vi "AlliGator Run FLI Dataset Python Function (API v1.1).vi"(7 "AlliGator Ctrl Refnums":T1, 8 "error in (no error)":errorcluster, 9 "Current Data":string, 10 "Python Function Info":T10={"Script Path"=path "", "Function Name"="", "Function Parent Menu"="", "API Version"="", "Function Input Parameters"=[], "Function Outputs"=[], "Function Doc String"="", "Function Display Name"="", "Function Target Type"=enum."Window Menu", "Function Target Window"="", "Parent Menu Location"="", "Item Menu Tag"="", "Is preceded by Separator"=FALSE}, 11 "Data Value Reference in":refnum<data-value>) -> (0 "error out":errorcluster, 1 "Message":string, 2 "Function Output Destination":string, 3 "Data Value Reference out":refnum<data-value>, 4 "Variant data out":variant)   [LabVIEW 2021, in "AlliGator Python Plugins.lvlib"]
doc: "Runs FLI Dataset python plugin function."
uses:
  AlliGator Python Plugins.lvlib
  Internal Variables/AlliGator Internal Variables v2.ctl
  <vilib>/vision/Image Controls.llb/IMAQ Image.ctl
  Internal Variables/AlliGator Gate Image Set.ctl
  Files/AlliGator FLI Dataset Type.ctl
  Files/AlliGator Data Series Type.ctl
  Dual-Channel Datasets/AlliGator Dataset Channel.ctl
  Settings/AlliGator Gate Arithmetic.ctl
  Source Image/AlliGator Displayed Image.ctl
  Image/Named ROI Description.ctl
  Phasor Graph/AlliGator Decay Metadata v3.ctl
  Decay Analysis/Decay Preprocessing/AlliGator Decay Background Subtraction Info.ctl
  Decay Analysis/Decay Preprocessing/AlliGator Baseline Subtraction Method.ctl
  Graphs/XY Graph/XY Graph Plot Shift Parameters.ctl
  Graphs/XY Graph/XY Graph Plot Shift Method.ctl
  Decay Analysis/Decay Preprocessing/AlliGator Decay Extrapolation Parameters.ctl
  Phasor/Calibration Phasor (m, phi).ctl
  Phasor/Phasor Reference Series.ctl
  Phasor/Phasor Calibration Map v2.ctl
  Phasor/Phasor (g, s).ctl
  Phasor Graph/AlliGator Raw Phasor Plot Data v5.ctl
  Phasor/Phasor Standard Deviation Options.ctl
  Phasor Plot/AlliGator Phasor Multi-Harmonic Data.ctl
  Phasor/Phasor Harmonic Data.ctl
  Decay Fit Parameter Map/AlliGator Decay Fit Options & Parameters v4.ctl
  Fits/IRF(X)PSED/Decay Fit Options v4.ctl
  Fits/Decay Convolution/Decay Model.ctl
  Fits/Residual Type.ctl
  Fits/IRF(X)PSED/Fit Weights Type v2.ctl
  Fits/Non-linear Fitting Method v2.ctl
  Fits/Fit Calculation Method.ctl
  Fits/Non-linear Fitting Algorithm.ctl
  Decay Analysis/Decay Fit/AlliGator Decay Fit Parameter Constraints 2.ctl
  Fits/IRF(X)PSED/Decay Fit Parameters In List.ctl
  Fits/IRF(X)PSED/MLE Baseline Offset Type.ctl
  Decay Analysis/Decay Preprocessing/AlliGator Decay Preprocessing Parameters.ctl
  Fits/IRF(X)PSED/Decay Fit Parameters & Derived Quantities List v2.ctl
  Fits/IRF(X)PSED/Decay Fit Result Constraint.ctl
  Decay Fit Parameter Map/AlliGator Parameter Maps Data.ctl
  AlliGator Python Function Information.ctl
  AlliGator Python Function Parameter Definition.ctl
  AlliGator Python Function Output Definition.ctl
  AlliGator Python Plugin Target Type.ctl
  Globals, Variables, Constants/AlliGator Variables List.ctl
  AlliGator Python Plugin Data v1.1.ctl
  API v1/AlliGator Python Plugin Image Data v1.ctl
  API v1/AlliGator Python Plugin Graph Data v1.ctl
  API v1/AlliGator Python Plugin Plot Data v1.ctl
  AlliGator Python Plugin Parameter Map Data v1.1.ctl
  Image/Image Point.ctl
  AlliGator Python Plugin FLI Dataset Data v1.1.ctl
  Parameter Map/AlliGator New Parameter Map Set Event Data.ctl
  <vilib>/Utility/error.llb/Error Cluster From Error Code.vi
  <vilib>/ErrorRing/Error Ring.xnode
  Globals, Variables, Constants/AlliGator Globals, Variables & Constants.lvlib
  Error/Error.lvlib
  Image/Image.lvlib
  Time/Time.lvlib
  Parameter Map/AlliGator Parameter Map.lvlib
  Strings/Strings.lvlib
  Phasor/Phasor.lvlib
  Decay Analysis/Decay Preprocessing/AlliGator Decay Preprocessing.lvlib
  Graphs/XY Graph/XY Graph Add-Ons.lvlib
  Phasor Graph/AlliGator Phasor Graph.lvlib
  Files/AlliGator Files.lvlib
  Phasor Plot/AlliGator Phasor Plot.lvlib
  Source Image/AlliGator Source Image.lvlib
  Fits/Fits.lvlib
  Decay Analysis/Decay Fit/AlliGator Decay Fit.lvlib
  Internal Variables/AlliGator Internal Variables.lvlib
  Settings/AlliGator Settings.lvlib
  Dual-Channel Datasets/AlliGator Dual-Channel Datasets.lvlib
  Decay Fit Parameter Map/AlliGator Decay Fit Parameter Map.lvlib
  GUI/AlliGator Registered Events Ctrl Refnums.ctl
  GUI/AlliGator GUI.lvlib
  GUI/AlliGator Dataset Ctrl Refnums.ctl
  Phasor/Phasor Calibration Type.ctl
  GUI/AlliGator Phasor Graph Ctrl Refnums.ctl
  GUI/AlliGator Phasor Plot Ctrl Refnums.ctl
  GUI/AlliGator State Indicator.ctl
  GUI/AlliGator Main Window Tabs.ctl
  GUI/AlliGator Other Ctrl Refnums.ctl
  Histograms/Histogram Bin Position.ctl
  Histograms/Histogram Window.lvlib
  Histograms/Histogram Bin Option.ctl
  Histograms/Linear Histogram Options.ctl
  GUI/AlliGator Image Histogram Control Refnums.ctl
  Decay Fit Parameter Map/AlliGator Decay Fit Map Control Refnums.ctl
  Parameter Map/AlliGator Parameter Map Control Refnums.ctl
  GUI/AlliGator Ctrl Refnums.ctl
panel:
  out "session out":refnum<k35>
  out "Function Parameters String":string
  # "see the AlliGator License on the block diagram (Ctrl+E or Window:Show Block Diagram)"
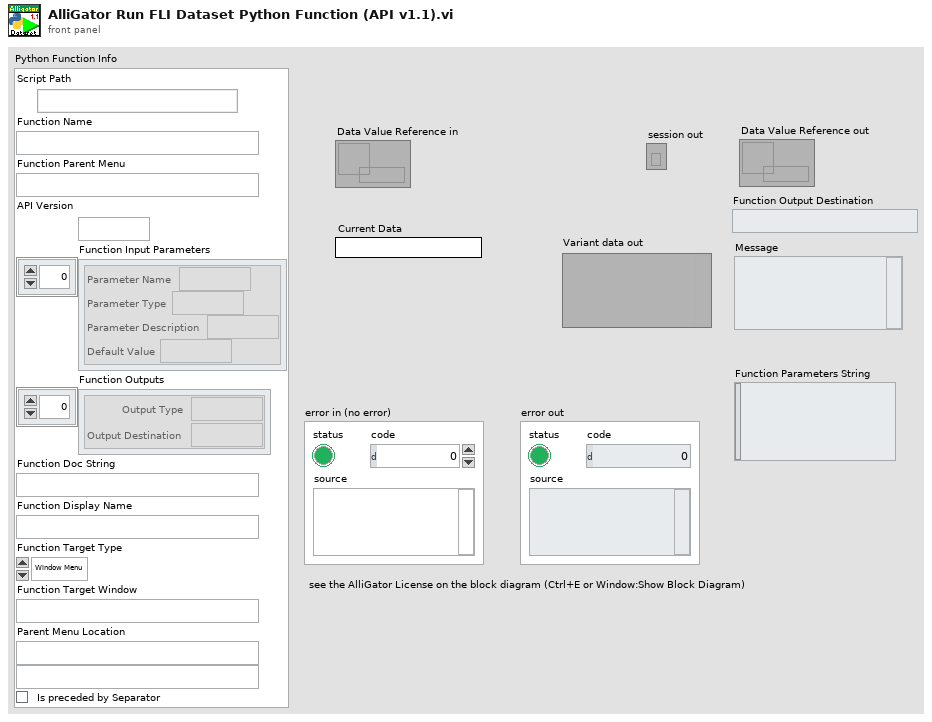
[diagram p1: front panel]
types:
  T1 = typedef "AlliGator GUI.lvlib/AlliGator Ctrl Refnums.ctl" = cluster{"Other AlliGator Ctrl Refnums":T2, "Phasor Plot Ctrl Refnums":T3, "Phasor Graph Ctrl Refnums":T4, "Dataset Control Refnums":T5, "Registered Events Ctrl Refnums":T6, "Image Histogram Ctrl Refnums":T7, "Decay Fit Map Ctrl Refnums":T8, "Parameter Map Ctrl Refnums":T9}
  T2 = typedef "AlliGator GUI.lvlib/AlliGator Other Ctrl Refnums.ctl" = cluster{"State Indicators":refnum<vi>, " Progress Bar":refnum<vi>, "Decay Graph Active":refnum<vi>, "Decay Statistics Bin":refnum<vi>, "Time Step":refnum<vi>, "Use File Timestamp":refnum<vi>, "Tab Control":refnum<vi>, "CPU":refnum<vi>, "Abort Fit":refnum<vi>, "Dataset File/Folder Path":refnum<vi>, "Abort ROI Creation":refnum<vi>, "Event LED":refnum<vi>, "Dataset File/Folder Path 2":refnum<vi>, "Dataset File/Folder Path 3":refnum<vi>, "Dataset File/Folder Path 4":refnum<vi>, "Dataset File/Folder Path 5":refnum<vi>, "Dataset File/Folder Path 6":refnum<vi>, "Dataset File/Folder Path 7":refnum<vi>, "Dataset File/Folder Path 8":refnum<vi>, "Dataset File/Folder Path 9":refnum<vi>, "Dataset File/Folder Path 10":refnum<vi>, "Dataset File/Folder Path 11":refnum<vi>}
  T3 = typedef "AlliGator GUI.lvlib/AlliGator Phasor Plot Ctrl Refnums.ctl" = cluster{"Phasor Ratio":refnum<vi>, "Modulus Lifetime":refnum<vi>, "Phasor at cursor (m, phi)":refnum<vi>, "Phase Lifetime":refnum<vi>, "Phasor at cursor (g, s)":refnum<vi>, "Phasor Plor Average Lifetime":refnum<vi>, "Phasor Plot Active":refnum<vi>, "Save Phasor Plot":refnum<vi>, "Image Overlay Color":refnum<vi>, "Phasor Plot Color Scale":refnum<vi>, "Reference 1 Button":refnum<vi>, "Reference 2 Button":refnum<vi>, "True Phasor Plot Value":refnum<vi>}
  T4 = typedef "AlliGator GUI.lvlib/AlliGator Phasor Graph Ctrl Refnums.ctl" = cluster{"Phasor Ratio":refnum<vi>, "Modulus Lifetime":refnum<vi>, "Phasor at cursor (m, phi)":refnum<vi>, "Phase Lifetime":refnum<vi>, "Phasor at cursor (g, s)":refnum<vi>, "Phasor Graph Average Lifetime":refnum<vi>, "Phasor Graph Active":refnum<vi>, "Save Phasor Graph":refnum<vi>, "Phasor Frame Slide":refnum<vi>, "Single Step Phasor":refnum<vi>, "Calibration Type":refnum<vi>, "Show Line":refnum<vi>, "Phase Lifetime 1":refnum<vi>, "Phase Lifetime 2":refnum<vi>, "Phasor Graph Frequency":refnum<vi>, "Phasor Reference 1 Control":refnum<vi>, "Phasor Reference 2 Control":refnum<vi>, "Calibration Lifetime":refnum<vi>, "Phase Lifetime SDV":refnum<vi>, "Average Lifetime SDV":refnum<vi>, "Phasor Ratio SDV":refnum<vi>, "Modulus Lifetime SDV":refnum<vi>}
  T5 = typedef "AlliGator GUI.lvlib/AlliGator Dataset Ctrl Refnums.ctl" = cluster{"Current Data":refnum<vi>, "Gate Image Slide":refnum<vi>, "Time Point Slide":refnum<vi>, "Current Time Stamp":refnum<vi>, "Save Image":refnum<vi>, "Displayed Image":refnum<vi>, "Overlay Mode":refnum<vi>, "Phasor Overlay Color":refnum<vi>, "Image Color Scale":refnum<vi>, "Use ROI as Search Area":refnum<vi>, "Source Image ROI Color":refnum<vi>, "True Pixel Value":refnum<vi>}
  T6 = typedef "AlliGator GUI.lvlib/AlliGator Registered Events Ctrl Refnums.ctl" = cluster{"Time Point Slider":refnum<vi>, "Phasor Plot Display Range":refnum<vi>, "Decay Graph":refnum<vi>, "Decay Statistics Graph":refnum<vi>, "Intensity Time Trace":refnum<vi>, "Phasor Graph":refnum<vi>, "Phasor Ratio Graph":refnum<vi>, "Lifetime Graph":refnum<vi>, "Phasor Plot Display":refnum<vi>, "Source Image Display":refnum<vi>, "Decay Fit Parameter Map Display Range":refnum<vi>, "Decay Fit Parameter Map Display":refnum<vi>, "Parameter Map Display Range":refnum<vi>, "Parameter Map Display":refnum<vi>, "Phasor Plot Display Range":refnum<vi>}
  T7 = typedef "AlliGator GUI.lvlib/AlliGator Image Histogram Control Refnums.ctl" = cluster{"Image Histogram":refnum<vi>, "Image Histogram Options":refnum<vi>, "Image Histogram Active":refnum<vi>, "Image Histogram Upper Percentile":refnum<vi>, "Image Histogram Lower Percentile":refnum<vi>, "Auto-Adjust Contrast":refnum<vi>}
  T8 = typedef "AlliGator Decay Fit Parameter Map.lvlib/AlliGator Decay Fit Map Control Refnums.ctl" = cluster{"Decay Fit Parameter Map Color Scale":refnum<vi>, "Decay Fit Parameter":refnum<vi>, "Max Parameter":refnum<vi>, "Min Parameter":refnum<vi>, "Decay Fit Parameter Map Display":refnum<vi>, "Decay Fit Parameter Map Display Range":refnum<vi>, "Decay Parameter Map X":refnum<vi>, "Decay Parameter Map Y":refnum<vi>, "Decay Parameter Map Value":refnum<vi>}
  T9 = typedef "AlliGator Parameter Map.lvlib/AlliGator Parameter Map Control Refnums.ctl" = cluster{"Parameter Map Color Scale":refnum<vi>, "Map Parameter":refnum<vi>, "Max Parameter":refnum<vi>, "Min Parameter":refnum<vi>, "Parameter Map Display":refnum<vi>, "Parameter Map Display Range":refnum<vi>, "Parameter Map Set":refnum<vi>, "Parameter Map X":refnum<vi>, "Parameter Map Y":refnum<vi>, "Parameter Map Value":refnum<vi>}
  T10 = typedef "AlliGator Python Plugins.lvlib/AlliGator Python Function Information.ctl" = cluster{"Script Path":path, "Function Name":string, "Function Parent Menu":string, "API Version":string, "Function Input Parameters":T11[], "Function Outputs":T12[], "Function Doc String":string, "Function Display Name":string, "Function Target Type":T13, "Function Target Window":string, "Parent Menu Location":string, "Item Menu Tag":string, "Is preceded by Separator":bool}
  T11 = typedef "AlliGator Python Plugins.lvlib/AlliGator Python Function Parameter Definition.ctl" = cluster{"Parameter Name":string, "Parameter Type":string, "Parameter Description":string, "Default Value":string}
  T12 = typedef "AlliGator Python Plugins.lvlib/AlliGator Python Function Output Definition.ctl" = cluster{"Output Type":string, "Output Destination":string}
  T13 = typedef "AlliGator Python Plugins.lvlib/AlliGator Python Plugin Target Type.ctl" = enum16{"Undefined", "Window Menu", "Object Menu"}
  T14 = typedef "AlliGator Python Plugins.lvlib/AlliGator Python Plugin Data v1.1.ctl" = cluster{"Image_Plugin_Data":T15, "Graph_Plugin_Data":T16, "Parameter_Map_Plugin_Data":T18, "FLI_Dataset_Plugin_Data":T20}
  T15 = typedef "AlliGator Python Plugins.lvlib/AlliGator Python Plugin Image Data v1.ctl" = cluster{"Image_Name":string, "Image":sgl[][]}
  T16 = typedef "AlliGator Python Plugins.lvlib/AlliGator Python Plugin Graph Data v1.ctl" = cluster{"Graph_Name":string, "Plots":T17[], "Reference_Decay":T17}
  T17 = typedef "AlliGator Python Plugins.lvlib/AlliGator Python Plugin Plot Data v1.ctl" = cluster{"Plot_Name":string, "X_Array":dbl[], "Y_Array":dbl[]}
  T18 = typedef "AlliGator Python Plugins.lvlib/AlliGator Python Plugin Parameter Map Data v1.1.ctl" = cluster{"Parameter_Names":string[], "Parameter_Flattened_Map":dbl[][], "Locations":T19[], "IRF_X":dbl[], "IRF_Y_Flattened_List":dbl[][], "X_Resolution":i32, "Y_Resolution":i32}
  T19 = typedef "Image.lvlib/Image Point.ctl" = cluster{"X":i32, "Y":i32}
  T20 = typedef "AlliGator Python Plugins.lvlib/AlliGator Python Plugin FLI Dataset Data v1.1.ctl" = cluster{"FLI_Dataset_Name":string, "Gate_Duration":dbl, "Gate_Separation":dbl, "Gate_Number":i32, "X_Size":i32, "Y_Size":i32, "Image_Data_List":T15[], "Mask_Image":u16[][], "Sum_Image":sgl[][], "Max_Image":sgl[][], "Min_Image":sgl[][]}
  T21 = typedef "AlliGator Globals, Variables & Constants.lvlib/AlliGator Variables List.ctl" = enum16{"---- GUI ----", "GUI:Initialization Status", "GUI:State Indicators Refnum", "GUI:Original AlliGator Menu Items", "GUI:Current Action Loop State", "GUI:Script in progress", "GUI:Playback", "GUI:Loop Playback", "GUI:Search ROI Used", "GUI:Search ROI", "Decay Graph Max Legend Size", "Intensity Graph Max Legend Size", "Decay Statistics Graph Max Legend Size", "Phasor Graph Max Legend Size", "Phasor Ratio Graph Max Legend Size", "Lifetime Graph Max Legend Size", "---- Files ----", "Files:Export Dataset Frames as Individual Files", "Files:Show Batch Export Help Balloons", "Files:Frames in Dataset", "Files:ptu File Frame Start Indices", "Files:Current Frame in Dataset", "Files:Current Frame Timestamp", "Files:Dataset Loaded", "Files:Dataset Metadata", "Files:Dataset Channel", "Files:Dataset Data Description", "Files:Background Dataset Metadata", "Files:Background Dataset Channel", "Files:Background Dataset Data Description", "Files:Background File Subtraction", "Files:Background File Path", "Files:Background File Pile-up Correction", "Files:Background File Pixel Well Capacity", "Files:Background File Scaling Factor", "Files:Current Dataset Load Settings", "Files:Dataset Path", "Files:ICCD-specific Information", "Files:Macrotime Gate Separation", "------ Python Plugins ------", "Python Plugins:Information", "Python Plugins:Python Session", "Python Plugins:Valid Python Session?", "---- Source Image ----", "Source Image:ROIs", "Source Image:Current ROI", "Source Image:ROI Event Refnum", "X_Source Image:Display Range", "X_Source Image:Palette Information", "X_Source Image:Type of Displayed Image", "X_Time Gate Slider", "Source Image:Palette List", "Source Image:Scale", "Source Image:ROI Overlay Color", "Source Image:Overlay to Erase", "Source Image:Is Displayed Image Accumulated", "Source Image:White Light Image Modified", "Source Image:Mask Image Modified", "---- Image Profile Window ----", "Image Profile:Window Event Refnum", "Image Profile:IntensityType", "Image Profile:Intensity Average Type", "Image Profile:Intensity-weighted SDV", "Image Profile:Box Profile Type", "Image Profile:Window Open", "Image Profile:Plotted Fit Parameter", "------ Phasor Graph -------", "Phasor Graph:Show Line", "---- Phasor Plot ---", "Phasor Plot:Parameters Changed", "Phasor Plot:FLI Dataset Modified since last Calculation", "Phasor Harmonics Data", "Selected Phasor Harmonics", "Phasor Harmonic Manager Event Refnum", "Phasor Plot:ROIs", "Phasor Plot:Current ROI", "Phasor Plot:ROI Event Refnum", "Phasor Plot:Image Reference Points", "Phasor Plot:Computed", "Phasor Plot:Palette Information", "Phasor Plot:Palette List", "Phasor Plot:Phasor Ratio Palette Information", "Phasor Plot:Phasor Ratio Palette List", "Phasor Plot:Image Scale", "Phasor Plot:Image Overlay to Erase", "Phasor Plot:Image Elements to Update", "Phasor Plot:Current Calculation Parameters", "Phasor Plot:Current Calibration Options", "Phasor Plot:Reset Cumulated Phasor Plot", "Phasor Plot:Reference 1", "Phasor Plot:Lifetime Reference 1", "Phasor Plot:Reference 1 Frequency", "Phasor Plot:Reference 2", "Phasor Plot:Lifetime Reference 2", "Phasor Plot:Reference 2 Frequency", "---- Decay Analysis ----", "Number of Selected Decays to Fit", "LS Fit Results", "LAR Fit Results", "BS Fit Results", "Last Decay Max - Min", "Best Fit Parameters", "Best Fit Parameter Names", "Actual Size X", "Actual Size Y", "Binning X", "Binning Y", "Actual # Gates", "Dataset Number", "Gates to...", "Gates Skipped", "Gates to keep", "Gate Step", "Gate Separation", "Reversed Gates", "Pile-up Correction", "Pixel Well Capacity", "Background Subtracted", "Background Subtraction Method", "Background Definition Range", "Background File (deprecated)", "Number of Dataset Accumulated", "Array of Accumulated Dataset Paths", "Do Averaged Datasets", "Destination File Path", "Process Plot Target", "Use 1/D as Phasor Frequency", "---- Decay Fit Parameter Map -----", "Decay Fit Parameter Map:Palette Information", "Decay Fit Parameter Map:Palette List", "Decay Fit Parameter Map:X Resolution", "Decay Fit Parameter Map:Y Resolution", "Decay Fit Parameter Map:Use Decay Fit Result Constraints", "Decay Fit Parameter Map:Decay Fit Result Constraints", "Decay Fit Parameter Map:Decay Fit Result Constraints Applied", "---- Parameter Map ----", "Parameter Map:Palette Information", "Parameter Map:Palette List", "------- Local Decay Window ---------", "Local Decay Graph Window:Event Refnum", "Local Decay Graph Window:Use normalized IRF for convolution", "----- Miscellaneous ----", "Misc:Skippable Dialog Windows Status"}
  T22 = typedef "AlliGator Parameter Map.lvlib/AlliGator New Parameter Map Set Event Data.ctl" = cluster{"New Parameter Set Name":string, "Parameter Map Names":string[]}
  T23 = typedef "AlliGator Internal Variables.lvlib/AlliGator Internal Variables v2.ctl" = cluster{"----------------------------- Images -----------------------------":u8, "Displayed Image":T24, "White Light Image":T24, "Mask Image":T24, "ROI Mask Image":T24, "Current Dataset Images 1":T25, "Background Dataset Images 1":T25, "Current Dataset Images 2":T25, "Background Dataset Images 2":T25, "Current Dataset Arithmetic Images":T25, "Accumulated Dataset Images 1":T25, "Accumulated Dataset Images 2":T25, "Accumulated Dataset Arithmetic Images":T25, "----------------------------- File Paths -----------------------------":u8, "Phasor Plot Image":T24, "Decay Fit Parameter Map Image":T24, "Parameter Map Image":T24, "Single Data Point Path":path, "White Light Image Path":path, "Mask Image Path":path, "Time-Series Folder":path, "[Time-Series Paths]":path[], "----------------------------- FLI Dataset -----------------------------":u8, "Current Dataset":i32, "Single Dataset Type":T26, "Current Folder":string, "AlliGator Data Series Type":T27, "# Datasets":i32, "Dual-Channel Dataset":bool, "Selected Channel Name":string, "Dataset Channel":T28, "Channel Arithmetic":T29, "Dual-Channel Background Dataset":bool, "Background Channel":T28, "Dual-Channel Accumulated Dataset":bool, "Start Time":dbl, "[Time-Series Timestamps]":dbl[], "[Intensity Corrections]":dbl[], "Time Series Script":bool, "Type of Displayed Image":T30, "Gate Image Slide":u16, "# Gates":i32, "ROIs":T31[], "----------------------------- Decays -----------------------------":u8, "ROI Decay":cluster{"t Array":dbl[], "I Array":dbl[]}, "Valid Decay":bool, "Decay  Metadata":T33, "Reference Decay Plot Name":string, "Reference Decay":cluster{"t Array":dbl[], "I Array":dbl[]}, "Decay Shift Plot":cluster{"Time Stamps":dbl[], "Decay Shifts":dbl[]}, "[Decays Max Values]":sgl[], "[Decays Min Values]":sgl[], "----------------------------- Calibration -----------------------------":u8, "Calibration Phasor":T39, "Calibration Phasor Series":T40, "Phasor Calibration Map":T41, "Calibration Map MD5 Digest":string, "----------------------------- Phasor Graph -----------------------------":u8, "Last Raw Phasor":T42, "Last Calibrated Phasor":T42, "Last Calibrated Phasor SDV":T42, "Phasor Graph:Phasor Plot":cluster{"g Array":dbl[], "s Array":dbl[]}, "Phasor Graph:Phasor SDV Plot":cluster{"g Array":dbl[], "s Array":dbl[]}, "[Phasor Graph:Raw Phasor Plots]":T43[], "Phasor Plot locked to Ref 1":i32, "[Phasor Plot(s) locked to Ref 1]":i32[], "[Phasor Plot(s) locked to Ref 2]":i32[], "[Pixel Phasors]":T42[], "----------------------------- Phasor Plot -----------------------------":u8, "[[Sum Image]]":dbl[][], "[[CSG Phasors]]":csg[][], "[[Valid Pixel?]]":bool[][], "[[Phasor Ratios]]":dbl[][], "[[Average Lifetimes]]":dbl[][], "Amplitude Weighted Average Lifetime":bool, "I/m/phi Dataset":cluster{"I/m/phi Dataset?":bool, "Base Frequency":dbl[unit], "Harmonic Orders":u8[]}, "Multi Phasor Plot Data":T45, "----------------------------- Decay Fit Parameter Map -----------------------------":u8, "Decay Fit Options & Parameters":T47, "Fit Options: Decay Preprocessing Parameters":T58, "Fit Options: Reference Decay":cluster{"t Array":dbl[], "I Array":dbl[]}, "Is Full Image Parameters Map":bool, "Is Single-Pixels Parameters Map":bool, "NLSF Parameters Map X Resolution":i32, "NLSF Parameters Map Y Resolution":i32, "[Single Decay Fit Parameters]":dbl[], "Fit Model":T49, "[[Multiple Decays Fit Parameters]]":dbl[][], "[[Multiple Decays Fit Parameter SDVs]]":dbl[][], "[[IRFs]]":dbl[][], "[ROI Descriptors]":T32[], "IRF Array Time Axis":dbl[], "Decay Array Time Axis":dbl[], "[Decay Fit Parameter Names]":T59[], "[Decay Sum]":dbl[], "Array of Decay Fit Result Constraints":T60[], "Selected ROIs Array":bool[], "----------------------------- Parameter Maps -----------------------------":u8, "[Map Set Names]":string[], "[Parameter Maps]":T61[], "[[User-defined Quantities]]":dbl[][], "User-defined Quantity":string}
  T24 = typedef "IMAQ Image.ctl" = refnum<image>
  T25 = typedef "AlliGator Internal Variables.lvlib/AlliGator Gate Image Set.ctl" = cluster{"SGL Gate Images":T24[], "SGL Sum Image":T24, "SGL Max Image":T24, "SGL Min Image":T24}
  T26 = typedef "AlliGator Files.lvlib/AlliGator FLI Dataset Type.ctl" = enum16{"HDF5 FLI Dataset", "Gate Image Folder", ".sdt FLI Dataset (Becker & Hickl)", ".ptu FLI Dataset (PicoQuant)", "SS1 FLI Dataset", "SS2 FLI Dataset", "I/m/phi Dataset", ".bin FLI Dataset (PicoQuant Binned)", ".bin FLI Dataset (Piccolo Binned)", ".mat FLI Dataset"}
  T27 = typedef "AlliGator Files.lvlib/AlliGator Data Series Type.ctl" = enum16{"Not a Supported Series", "Gate Images Folder Series", "SwissSPAD 2 Dataset Series", "B&H FLI Dataset Series", "PicoQuant PTU FLI Dataset Series", "PicoQuant BIN FLI Dataset Series", "Piccolo hist BIN FLI Dataset Series", "HDF5 FLI Dataset Series"}
  T28 = typedef "AlliGator Dual-Channel Datasets.lvlib/AlliGator Dataset Channel.ctl" = enum16{"G2", "INT"}
  T29 = typedef "AlliGator Settings.lvlib/AlliGator Gate Arithmetic.ctl" = enum16{"None", "INT-G2", "G2/INT*<INT>", "(1 - G2/INT)*<INT>"}
  T30 = typedef "AlliGator Source Image.lvlib/AlliGator Displayed Image.ctl" = enum16{"Single Gate", "Sum of All Gates", "Max of All Gates", "Min of All Gates", "-", "White Ligth Image", "Mask Image"}
  T31 = typedef "Image.lvlib/Named ROI Description.ctl" = cluster{"ROI Descriptor":T32, "ROI Name":string, "Overlay Color":u32}
  T32 = typedef "ROI Descriptor" = cluster{"Global Rectangle":i32[], "Contours":cluster{"ID":enum32{"External", "Internal"}, "Type":u32, "Coordinates":i32[]}[]}
  T33 = typedef "AlliGator Phasor Graph.lvlib/AlliGator Decay Metadata v3.ctl" = cluster{"ROI Descriptor":T32, "ROI Center":cluster{"X":i32, "Y":i32}, "Decay Background Subtraction Info":T34, "Decay Reverted":bool, "Decay Smoothened":bool, "Decay Straightened":bool, "Fitted Tau (Decay Straightening)":dbl, "Decay Shift Parameters":T36, "Decay Shifted":bool, "Decay Extrapolated":bool, "Decay Extrapolation Parameters":T38, "Decay Normalized":bool, "Fold Decay":bool, "# Folds":u32}
  T34 = typedef "AlliGator Decay Preprocessing.lvlib/AlliGator Decay Background Subtraction Info.ctl" = cluster{"Laser Period":dbl[unit], "Gate Duration":dbl[unit], "Baseline Subtraction Method":T35, "Background Definition Range":cluster{"Min Gate":dbl[unit], "Max Gate":dbl[unit]}, "Total Intensity w/o Bkgd Subtraction":dbl, "Bkgd-subtracted Intensity (exp)":dbl, "# Data Points":i32, "Background/Gate":dbl, "Fitted Lifetime":dbl[unit], "Bkgd-subtracted Intensity (theo)":dbl}
  T35 = typedef "AlliGator Decay Preprocessing.lvlib/AlliGator Baseline Subtraction Method.ctl" = enum16{"Mean", "Min", "Square Gated Single-Exponential", "File", "Constant"}
  T36 = typedef "XY Graph Add-Ons.lvlib/XY Graph Plot Shift Parameters.ctl" = cluster{"Type":T37, "Shift":dbl[unit], "Threshold":dbl, "Rotate":bool}
  T37 = typedef "XY Graph Add-Ons.lvlib/XY Graph Plot Shift Method.ctl" = enum16{"Default", "CFD", "Threshold", "Cross-Correlation"}
  T38 = typedef "AlliGator Decay Preprocessing.lvlib/AlliGator Decay Extrapolation Parameters.ctl" = cluster{"Additional Points":u32, "Head Fraction":dbl, "Fitted Tau":dbl, "Use Periodicity":bool, "Use Cursors":bool, "Tail Fraction":dbl}
  T39 = typedef "Phasor.lvlib/Calibration Phasor (m, phi).ctl" = cluster{"m":dbl, "phi":dbl, "Phasor Frequency":dbl[unit], "Reference Lifetime":dbl[unit]}
  T40 = typedef "Phasor.lvlib/Phasor Reference Series.ctl" = cluster{"m Array":dbl[], "phi Array":dbl[], "Phasor Frequency":dbl[unit], "Calibration Lifetime":dbl[unit]}
  T41 = typedef "Phasor.lvlib/Phasor Calibration Map v2.ctl" = cluster{"Phasor Frequency":dbl[unit], "Calibration Lifetime":dbl[unit], "ROI Centers":cluster{"X":i32, "Y":i32}[], "ROI Descriptors":T32[], "Map Resolution X":i32, "Map Resolution Y":i32, "z Array":cdb[]}
  T42 = typedef "Phasor.lvlib/Phasor (g, s).ctl" = cluster{"g":dbl, "s":dbl}
  T43 = typedef "AlliGator Phasor Graph.lvlib/AlliGator Raw Phasor Plot Data v5.ctl" = cluster{"Phasor Plot Name":string, "Raw Phasor Plot":T42[], "Phasor Frequency":dbl[unit], "[Decay Metadata]":T33[], "Raw Phasor Plot SDV":T42[], "Phasor SDV Options":T44, "[Calibration Phasor]":T39[], "Intensity Array":dbl[]}
  T44 = typedef "Phasor.lvlib/Phasor Standard Deviation Options.ctl" = cluster{"Compute Estimated SDV":bool, "# Replicas":u32, "Use Estimated Average Phasor":bool}
  T45 = typedef "AlliGator Phasor Plot.lvlib/AlliGator Phasor Multi-Harmonic Data.ctl" = cluster{"Base Frequency":dbl[unit], "# Harmonics":u8, "Harmonic Orders":u8[], "Phasor Plot Settings Checksum":u64, "Phasor Harmonic Data Array":T46[]}
  T46 = typedef "Phasor.lvlib/Phasor Harmonic Data.ctl" = cluster{"Phasor Harmonic Name":string, "Phasor Plot Settings Checksum":u64, "Phasor Frequency":dbl[unit], "Base Frequency":dbl[unit], "Harmonic Order":u8, "Phasor Plot Parameters":string, "Phasor Array [[CSG]]":csg[][], "Dataset File Path":path}
  T47 = typedef "AlliGator Decay Fit Parameter Map.lvlib/AlliGator Decay Fit Options & Parameters v4.ctl" = cluster{"SYNC Period":dbl[unit], "Fit Options":T48, "Fit Parameter Constraints":T55[], "MLE Baseline Offset":dbl, "MLE Baseline Offset Type":T57}
  T48 = typedef "Fits.lvlib/Decay Fit Options v4.ctl" = cluster{"Show Fit Residuals":bool, "Fit Model":T49, "Residual Type":T50, "Max Decay Percentile":dbl, "Min Decay Percentile":dbl, "Show Full Decay":bool, "Weights":T51, "Fitting Method":T52, "Compute Parameter Uncertainties":bool, "Periodic Boundaries":bool, "Model Calculation":T53, "Period":dbl[unit], "Termination Criteria":cluster{"Max Iterations":i32, "Max Function Calls":i32, "Max Time":dbl[unit], "Function Tolerance":dbl, "Parameter Tolerance":dbl, "Gradient Tolerance":dbl, "Min Lambda":dbl, "Max Lambda":dbl, "Initial Tick Count":u32}, "Offset Resolution":dbl[unit], "Use Local IRF":bool, "Fitting Algorithm":T54, "Show Confidence Interval ":bool, "Confidence Level":dbl}
  T49 = typedef "Fits.lvlib/Decay Model.ctl" = enum16{"1-Exponential", "2-Exponentials"}
  T50 = typedef "Fits.lvlib/Residual Type.ctl" = enum16{"Standard", "Normalized", "Reduced"}
  T51 = typedef "Fits.lvlib/Fit Weights Type v2.ctl" = enum16{"Unweighted", "1/Variance (Neyman)", "1/Variance (Pearson)", "Best of All"}
  T52 = typedef "Fits.lvlib/Non-linear Fitting Method v2.ctl" = enum16{"Least Square", "Least Absolute Residual", "Bisquare", "MLE", "-", "Best of All"}
  T53 = typedef "Fits.lvlib/Fit Calculation Method.ctl" = enum16{"Simulation", "Convolution", "Integration"}
  T54 = typedef "Fits.lvlib/Non-linear Fitting Algorithm.ctl" = enum16{"Levenberg-Marquardt", "Trust-Region Dogleg"}
  T55 = typedef "AlliGator Decay Fit.lvlib/AlliGator Decay Fit Parameter Constraints 2.ctl" = cluster{"Fit Parameter":T56, "Min Value":dbl, "Max Value":dbl, "Global":bool, "Used":bool}
  T56 = typedef "Fits.lvlib/Decay Fit Parameters In List.ctl" = enum16{"Offset", "Baseline", "A_1", "tau_1", "A_2", "tau_2"}
  T57 = typedef "Fits.lvlib/MLE Baseline Offset Type.ctl" = enum32{"Absolute", "Percentage"}
  T58 = typedef "AlliGator Decay Preprocessing.lvlib/AlliGator Decay Preprocessing Parameters.ctl" = cluster{"Background Subtraction":bool, "Straighten Decay":bool, "Reverse Gates":bool, "1-Normalized Decay":bool, "Smoothen Decay":bool, "Smoothing Parameter":dbl, "Shift Decay":bool, "Decay Shift Parameters":T36, "Extrapolate Decay":bool, "Additional Points":u32, "Head Fraction":dbl, "Pixel-Normalize Decay":bool, "Use Periodicity":bool, "Use Cursors":bool, "Tail Fraction":dbl, "Use Decay Pre-Processing":bool, "Fold Decay":bool, "# Folds":u32, "[0-1]-Normalized Decay":bool}
  T59 = typedef "Fits.lvlib/Decay Fit Parameters & Derived Quantities List v2.ctl" = enum16{"Offset", "Baseline", "A_1", "tau_1", "A_2", "tau_2", "<tau>_a", "f1_a", "f2_a", "<tau>_i", "f1_i", "f2_i", "-", "R^2", "Chi^2"}
  T60 = typedef "Fits.lvlib/Decay Fit Result Constraint.ctl" = cluster{"Fit Parameter":enum16{"Offset", "Baseline", "A_1", "tau_1", "A_2", "tau_2", "<tau>_a", "f1_a", "f2_a", "<tau>_i", "f1_i", "f2_i", "-", "R^2", "Chi^2", "Max Relative Residual", "<Residual ACF>", "Residual ACF SDV", "tau_2/tau_1"}, "Min Value":dbl, "Max Value":dbl, "Use Constraint":bool}
  T61 = typedef "AlliGator Decay Fit Parameter Map.lvlib/AlliGator Parameter Maps Data.ctl" = cluster{"Map Set Name":string, "[Parameter Names]":string[], "[[Parameters]]":dbl[][], "[[Parameter SDVs]]":dbl[][], "Decay Array Time Axis":dbl[], "[[IRFs]]":dbl[][], "IRF Array Time Axis":dbl[], "X Resolution":i32, "Y Resolution":i32, "Intensity Array":dbl[]}
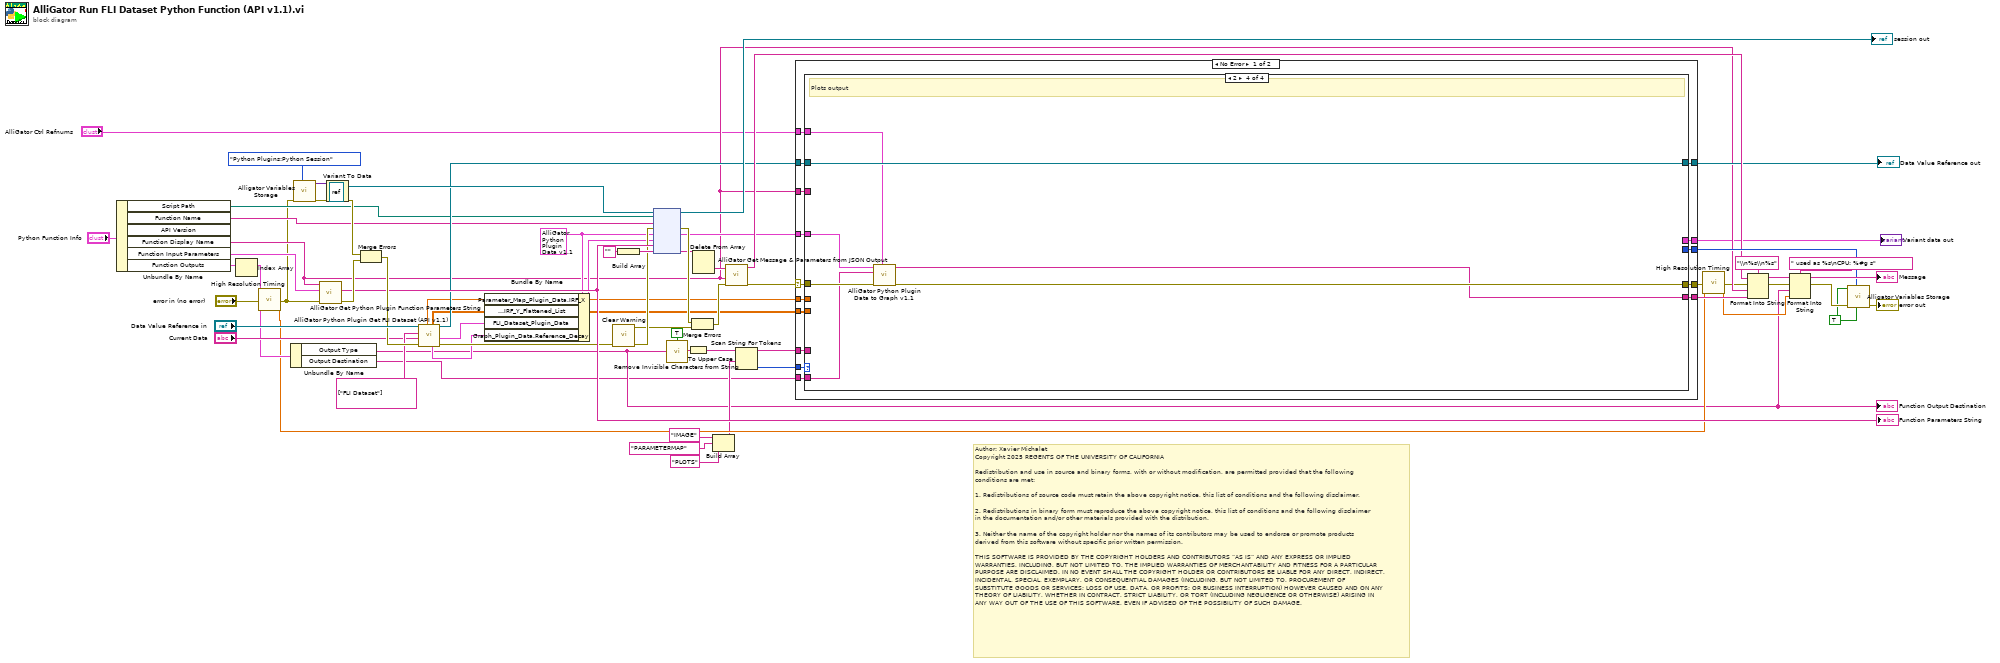
[diagram p0: block diagram]
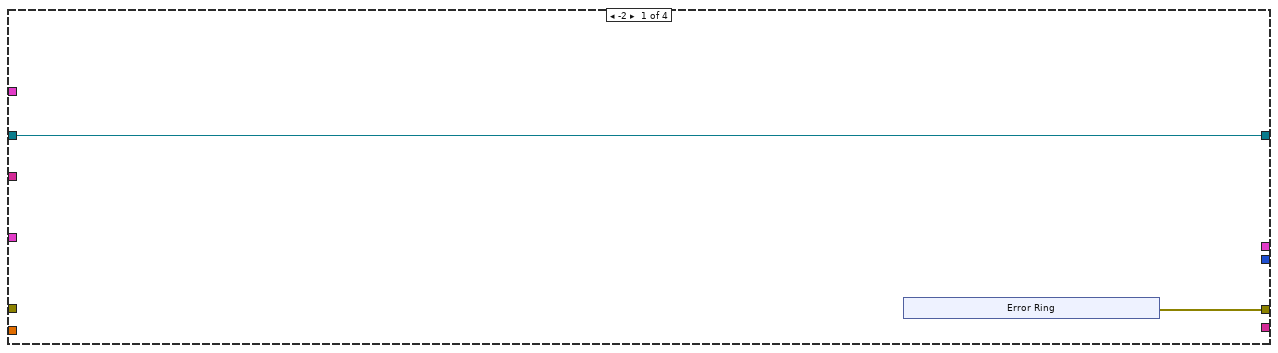
[diagram p2: hidden frame]
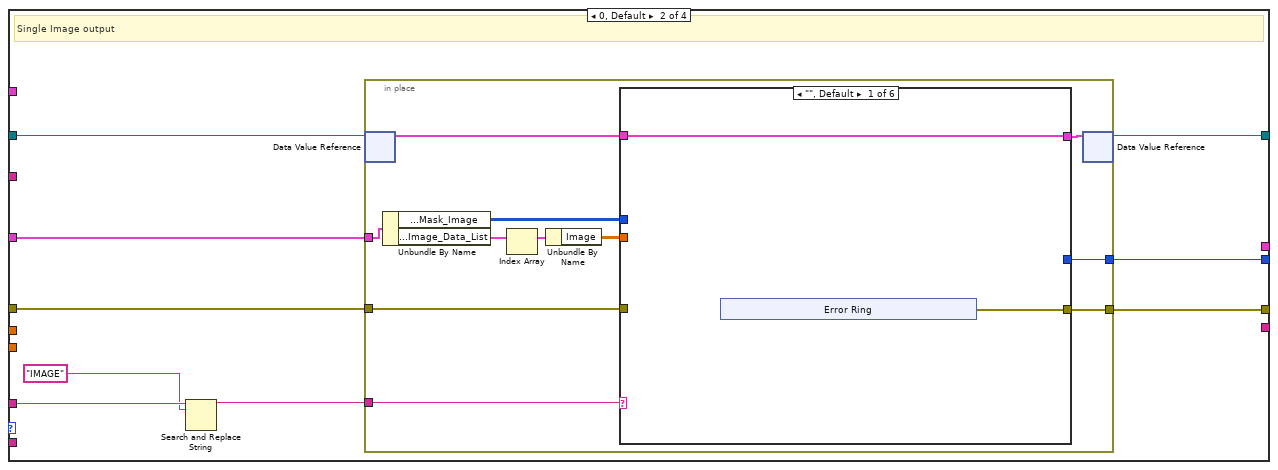
[diagram p3: hidden frame]
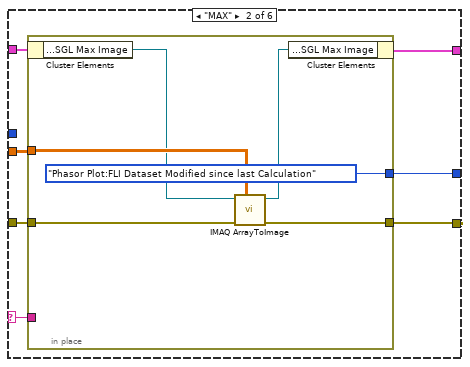
[diagram p4: hidden frame]
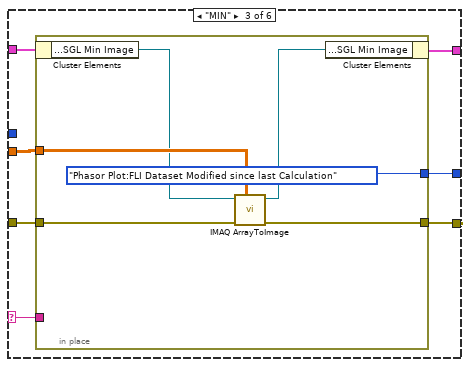
[diagram p5: hidden frame]
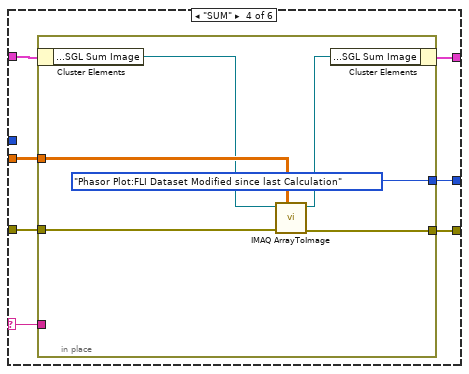
[diagram p6: hidden frame]
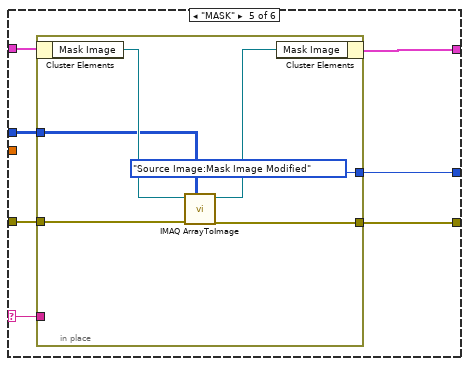
[diagram p7: hidden frame]
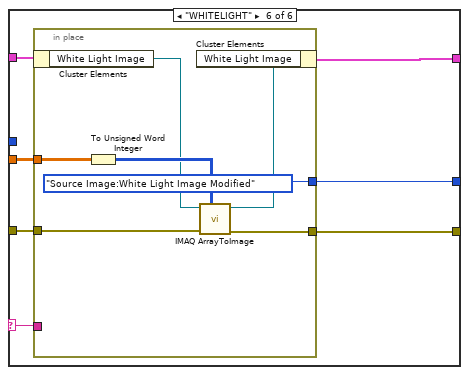
[diagram p8: hidden frame]
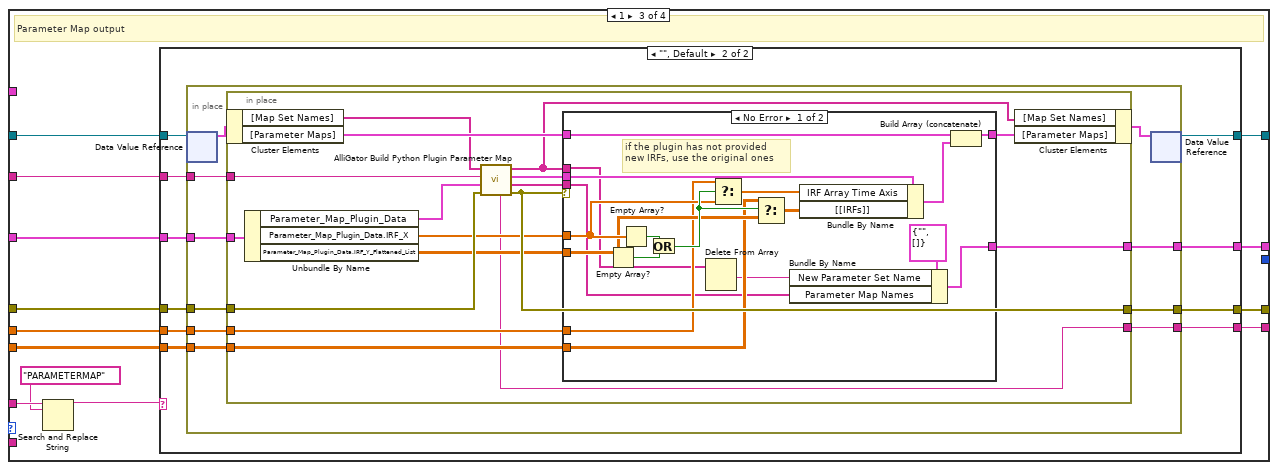
[diagram p9: hidden frame]
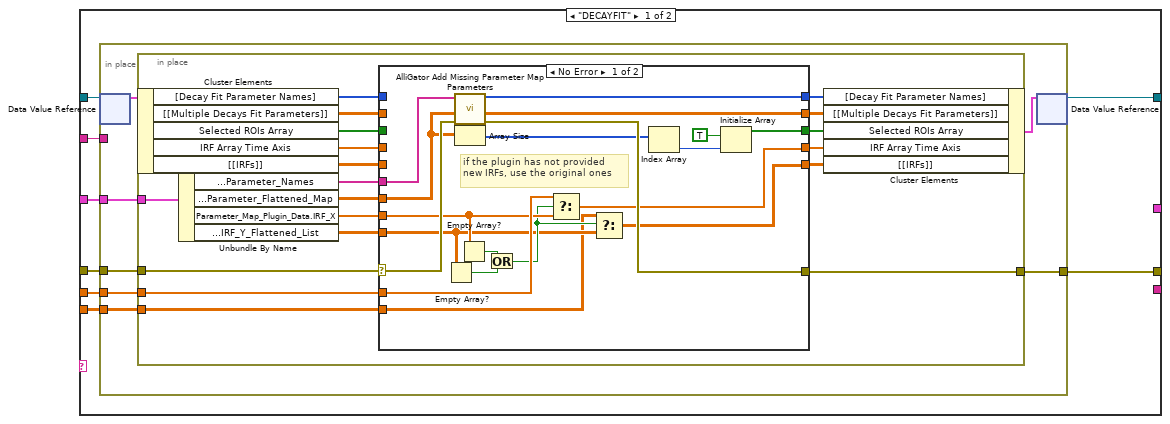
[diagram p10: hidden frame]
diagram:
  w27 = T14 {"Image_Plugin_Data"={"Image_Name"="", "Image"=[]}, "Graph_Plugin_Data"={"Graph_Name"="", "Plots"=[], "Reference_Decay"={"Plot_Name"="", "X_Array"=[], "Y_Array"=[]}}, "Parameter_Map_Plugin_Data"={"Parameter_Names"=[], "Parameter_Flattened_Map"=[], "Locations"=[], "IRF_X"=[], "IRF_Y_Flattened_List"=[], "X_Resolution"=0, "Y_Resolution"=0}, "FLI_Dataset_Plugin_Data"={"FLI_Dataset_Name"="", "Gate_Duration"=0.0, "Gate_Separation"=0.0, "Gate_Number"=0, "X_Size"=0, "Y_Size"=0, "Image_Data_List"=[], "Mask_Image"=[], "Sum_Image"=[], "Max_Image"=[], "Min_Image"=[]}} ("Plugin_Data")
  w51 = TRUE ("Get(F)/Set")
  # "Author: Xavier Michalet\nCopyright 2025 REGENTS OF THE UNIVERSITY OF CALIFORNIA\n\nRedistribution and use in source and binary forms, with or without modification, are permitted provided that the following conditions are met:\n\n1. Redistributions of source code must retain the above copyright notice, this list of conditions and the following disclaimer.\n\n2. Redistributions in binary form must reproduce the above copyright notice, this list of conditions and the following disclaimer in the documentation and/or other materials provided with the distribution.\n\n3. Neither the name of the copyright holder nor the names of its contributors may be used to endorse or promote products derived from this software without specific prior written permission.\n\nTHIS SOFTWARE IS PROVIDED BY THE COPYRIGHT HOLDERS AND CONTRIBUTORS “AS IS” AND ANY EXPRESS OR IMPLIED WARRANTIES, INCLUDING, BUT NOT LIMITED TO, THE IMPLIED WARRANTIES OF MERCHANTABILITY AND FITNESS FOR A PARTICULAR PURPOSE ARE DISCLAIMED. IN NO EVENT SHALL THE COPYRIGHT HOLDER OR CONTRIBUTORS BE LIABLE FOR ANY DIRECT, INDIRECT, INCIDENTAL, SPECIAL, EXEMPLARY, OR CONSEQUENTIAL DAMAGES (INCLUDING, BUT NOT LIMITED TO, PROCUREMENT OF SUBSTITUTE GOODS OR SERVICES; LOSS OF USE, DATA, OR PROFITS; OR BUSINESS INTERRUPTION) HOWEVER CAUSED AND ON ANY THEORY OF LIABILITY, WHETHER IN CONTRACT, STRICT LIABILITY, OR TORT (INCLUDING NEGLIGENCE OR OTHERWISE) ARISING IN ANY WAY OUT OF THE USE OF THIS SOFTWARE, EVEN IF ADVISED OF THE POSSIBILITY OF SUCH DAMAGE."
  n1 = Unbundle By Name("Python Function Info") -> ("Script Path"=w23:path, "Function Name"=w22:string, "Function Display Name"=w21:string, "Function Input Parameters"=w49:T11[], "Function Outputs"=w33:T12[])  [unwired: 1 out]
  n2 = Index Array(array=w33) -> (element=w32:T12)  [unwired: 1 in]
  n3 = call "High Resolution Timing.vi"("Error In"="error in (no error)") -> ("elapsed (relative) seconds"=w15:dbl, "Error Out"=w17:errorcluster)  [unwired: 16 in, 1 out]
  n4 = Unbundle By Name(w32) -> ("Output Type"=w6:string, "Output Destination"=w2:string)
  "Function Output Destination" <- w6
  n5 = call "Alligator Variables Storage.vi"("AlliGator Variable"=AlliGator_Variables_List."Python Plugins:Python Session" ("Alligator Variable"), "Error In"=w17) -> ("Error Out"=w65:errorcluster, "Data out"=w63:variant)  [unwired: 7 in, 1 out]
  n6 = call "AlliGator Get Python Plugin Function Parameters String.vi"("error in (no error)"=w17, "Function Parameters"=w49, "Function Display Name"=w21) -> ("error out"=w67:errorcluster, "Function Parameters JSON String"=w41:string)  [unwired: 6 in, 1 out]
  "Function Parameters String" <- w41
  n7 = Variant To Data(error in=w65, type=refnum<k35> refnum ("session in"), Variant=w63) -> (data=w61:refnum<k35>, error out=w64:errorcluster)
  n8 = Merge Errors(w64, w67) -> (w42:errorcluster)
  n9 = call "AlliGator Python Plugin Get FLI Dataset (API v1.1).vi"("error in (no error)"=w42, "Current Data"="Current Data", "AlliGator Parameter Names Not Found"=string[] ["FLI Dataset"], "Data Value Reference in"="Data Value Reference in") -> ("error out"=w31:errorcluster, "FLI_Dataset_Data"=w25:T20, "Data Value Reference out"=w40:refnum<data-value>, "Reference Decay"=w24:T17, "[[IRFs]]"=w18:dbl[][], "IRF Array Time Axis"=w19:dbl[])  [unwired: 1 in, 1 out]
  n10 = Bundle By Name(cluster=w27, "Parameter_Map_Plugin_Data.IRF_X"=w19, "Parameter_Map_Plugin_Data.IRF_Y_Flattened_List"=w18, "FLI_Dataset_Plugin_Data"=w25, "Graph_Plugin_Data.Reference_Decay"=w24) -> (w26:T14)
  n11 = call "Clear Warning.vi"("error in (no error)"=w31) -> ("cleared warning or error dup"=w30:errorcluster, "error in (dup)"=w28:errorcluster)  [unwired: 9 in]
  n12 = Build Array("") -> (w34:string[])
  n13 = node(w61, w23, w22, w30, w27, w26, w41, w34) -> (→"session out":refnum<k35>, w46:errorcluster, w36:T14, w44:string[])  [unwired: 2 in, 2 out]
  n14 = call "Remove Invisible Characters from String.vi"("Remove Line Feed. etc (F)"=TRUE, "String"=w6) -> ("result string"=w5:string)  [unwired: 2 in]
  n15 = To Upper Case(1:w5) -> (0:w4:string)
  n16 = Merge Errors(w46, w28) -> (w29:errorcluster)
  n17 = Delete From Array(array=w44) -> (deleted portion=w47:string)  [unwired: 2 in, 1 out]
  n18 = Build Array("IMAGE" ("search string"), "PARAMETERMAP" ("search string"), "PLOTS" ("search string")) -> (w9:string[])
  n19 = call "AlliGator Get Message & Parameters from JSON Output.vi"("error in (no error)"=w29, "Function Display Name"=w21, "<JSON>"=w47) -> ("error out"=w45:errorcluster, "Notebook Message"=w48:string)  [unwired: 7 in]
  n20 = Scan String For Tokens(7:w9, 9:w4) -> (0:w8:i32, 3:w7:string)  [unwired: 4 in, 2 out]
  n21 = case shown="No Error" w45 {
    selector: w45 -> [w82 w318]
    tunnel: [w84 w318] -> w69
    tunnel: [w83 _] -> w52
    tunnel: w40 -> [w81 w317]
    tunnel: [w80 w317] -> w39
    tunnel: w36 -> [w79 _]
    tunnel: w21 -> [w78 _]
    tunnel: [w77 _] -> w20
    tunnel: w19 -> [w76 _]
    tunnel: w18 -> [w75 _]
    tunnel: [w74 _] -> w13
    tunnel: w8 -> [w73 _]
    tunnel: w7 -> [w72 _]
    tunnel: w2 -> [w71 _]
    tunnel: "AlliGator Ctrl Refnums" -> [w70 _]
    frame No Error {
      n22 = case shown="2" w73 {
        tunnel: [w86 w99 w193 w315] -> w84
        tunnel: [_ w98 _ _] -> w83
        tunnel: w82 -> [_ w97 w192 w315]
        tunnel: w81 -> [w85 w96 w195 w316]
        tunnel: [w85 w95 w194 w316] -> w80
        tunnel: w79 -> [_ w94 w191 w314]
        tunnel: w78 -> [_ _ w190 _]
        tunnel: [_ _ w189 w312] -> w77
        tunnel: w76 -> [_ _ w188 _]
        tunnel: w75 -> [_ _ w187 _]
        tunnel: [_ _ w186 _] -> w74
        tunnel: w72 -> [_ w93 w185 _]
        tunnel: w71 -> [_ _ _ w313]
        tunnel: w70 -> [_ _ _ w311]
        frame -2 {
          n23 = xnode "Error Ring"() -> ("error out"=w86:errorcluster)
        }
        frame 0, Default {
          # "Single Image output"
          n24 = Search and Replace String(input string=w93, search string="IMAGE") -> (result string=w91:string)  [unwired: 6 in, 3 out]
          n25 = in-place {
            in-place-border: [w110] -> w99
            in-place-border: [w109] -> w98
            in-place-border: w97 -> [w108]
            in-place-border: w94 -> [w105]
            in-place-border: w91 -> [w100]
            n26 = in-place-dvr #1(w96) -> (w107:T23)  [unwired: 1 out]
            n27 = Unbundle By Name(w105) -> ("FLI_Dataset_Plugin_Data.Mask_Image"=w101:u16[][], "FLI_Dataset_Plugin_Data.Image_Data_List"=w104:T15[])
            n28 = Index Array(array=w104) -> (element=w103:T15)  [unwired: 1 in]
            n29 = Unbundle By Name(w103) -> ("Image"=w102:sgl[][])
            n30 = case shown="\"\", Default" w100 {
              selector: w100 -> [_ w119 w132 w146 w158 w171]
              tunnel: w107 -> [w112 w123 w136 w149 w162 w175]
              tunnel: w102 -> [_ w122 w135 w144 _ w174]
              tunnel: [w112 w121 w134 w148 w161 w173] -> w106
              tunnel: [w111 w120 w133 w147 w160 w172] -> w110
              tunnel: w108 -> [_ w118 w131 w145 w159 w170]
              tunnel: [_ w117 w130 w143 w157 w169] -> w109
              tunnel: w101 -> [_ _ _ _ w156 _]
              frame "", Default {
                n31 = xnode "Error Ring"() -> ("error out"=w111:errorcluster)
              }
              frame "MAX" {
                n32 = in-place {
                  in-place-border: w122 -> [w128]
                  in-place-border: w118 -> [w126]
                  in-place-border: [w127] -> w120
                  in-place-border: w119 -> [_]
                  in-place-border: [AlliGator_Variables_List."Phasor Plot:FLI Dataset Modified since last Calculation" ("Alligator Variable")] -> w117
                  n33 = in-place-cluster #2(w123) -> ("Current Dataset Images 1.SGL Max Image"=w124:T24)
                  n34 = call "IMAQ ArrayToImage"("Image Pixels (Float)"=w128, "error in (no error)"=w126, "Image"=w124) -> ("error out"=w127:errorcluster, "Image Out"=w129:T24)  [unwired: 7 in]
                  n35 = in-place-cluster #2("Current Dataset Images 1.SGL Max Image"=w129) -> (w121:T23)
                }
              }
              frame "MIN" {
                n36 = in-place {
                  in-place-border: w135 -> [w141]
                  in-place-border: w131 -> [w139]
                  in-place-border: [w140] -> w133
                  in-place-border: w132 -> [_]
                  in-place-border: [AlliGator_Variables_List."Phasor Plot:FLI Dataset Modified since last Calculation" ("Alligator Variable")] -> w130
                  n37 = in-place-cluster #3(w136) -> ("Current Dataset Images 1.SGL Min Image"=w137:T24)
                  n38 = call "IMAQ ArrayToImage"("Image Pixels (Float)"=w141, "error in (no error)"=w139, "Image"=w137) -> ("error out"=w140:errorcluster, "Image Out"=w142:T24)  [unwired: 7 in]
                  n39 = in-place-cluster #3("Current Dataset Images 1.SGL Min Image"=w142) -> (w134:T23)
                }
              }
              frame "SUM" {
                n40 = in-place {
                  in-place-border: w144 -> [w154]
                  in-place-border: [w153] -> w147
                  in-place-border: w146 -> [_]
                  in-place-border: w145 -> [w151]
                  in-place-border: [AlliGator_Variables_List."Phasor Plot:FLI Dataset Modified since last Calculation" ("Alligator Variable")] -> w143
                  n41 = in-place-cluster #4(w149) -> ("Current Dataset Images 1.SGL Sum Image"=w150:T24)
                  n42 = call "IMAQ ArrayToImage"("Image Pixels (Float)"=w154, "error in (no error)"=w151, "Image"=w150) -> ("error out"=w153:errorcluster, "Image Out"=w155:T24)  [unwired: 7 in]
                  n43 = in-place-cluster #4("Current Dataset Images 1.SGL Sum Image"=w155) -> (w148:T23)
                }
              }
              frame "MASK" {
                n44 = in-place {
                  in-place-border: [w167] -> w160
                  in-place-border: w159 -> [w165]
                  in-place-border: w158 -> [_]
                  in-place-border: [AlliGator_Variables_List."Source Image:Mask Image Modified" ("Alligator Variable")] -> w157
                  in-place-border: w156 -> [w163]
                  n45 = in-place-cluster #5(w162) -> ("Mask Image"=w166:T24)
                  n46 = call "IMAQ ArrayToImage"("Image Pixels (U16)"=w163, "error in (no error)"=w165, "Image"=w166) -> ("error out"=w167:errorcluster, "Image Out"=w168:T24)  [unwired: 7 in]
                  n47 = in-place-cluster #5("Mask Image"=w168) -> (w161:T23)
                }
              }
              frame "WHITELIGHT" {
                n48 = in-place {
                  in-place-border: w174 -> [w181]
                  in-place-border: [w180] -> w172
                  in-place-border: w171 -> [_]
                  in-place-border: w170 -> [w177]
                  in-place-border: [AlliGator_Variables_List."Source Image:White Light Image Modified" ("Alligator Variable")] -> w169
                  n49 = in-place-cluster #6(w175) -> ("White Light Image"=w176:T24)
                  n50 = To Unsigned Word Integer(number=w181) -> (unsigned 16bit integer=w179:u16[][])
                  n51 = call "IMAQ ArrayToImage"("Image Pixels (U16)"=w179, "error in (no error)"=w177, "Image"=w176) -> ("error out"=w180:errorcluster, "Image Out"=w182:T24)  [unwired: 7 in]
                  n52 = in-place-cluster #6("White Light Image"=w182) -> (w173:T23)
                }
              }
            }
            n53 = in-place-dvr #1(w106) -> (w95:refnum<data-value>)  [unwired: 1 out]
          }
        }
        frame 1 {
          # "Parameter Map output"
          n54 = Search and Replace String(input string=w185, search string="PARAMETERMAP") -> (result string=w183:string)  [unwired: 6 in, 3 out]
          n55 = case shown="\"\", Default" w183 {
            tunnel: w195 -> [w203 w264]
            tunnel: [w202 w263] -> w194
            tunnel: [w199 w260] -> w193
            tunnel: w192 -> [w200 w261]
            tunnel: w191 -> [w201 w262]
            tunnel: w190 -> [w196 w259]
            tunnel: [_ w258] -> w189
            tunnel: w188 -> [w198 w257]
            tunnel: w187 -> [w197 w256]
            tunnel: [_ w255] -> w186
            frame "DECAYFIT" {
              n56 = in-place {
                in-place-border: w201 -> [w209]
                in-place-border: w200 -> [w207]
                in-place-border: [w206] -> w199
                in-place-border: w198 -> [w205]
                in-place-border: w197 -> [w204]
                in-place-border: w196 -> [_]
                n57 = in-place-dvr #7(w203) -> (w210:T23)  [unwired: 1 out]
                n58 = in-place {
                  in-place-border: w209 -> [w229]
                  in-place-border: w207 -> [w225]
                  in-place-border: [w224] -> w206
                  in-place-border: w205 -> [w221]
                  in-place-border: w204 -> [w217]
                  n59 = in-place-cluster #8(w210) -> ("[Decay Fit Parameter Names]"=w215:T59[], "[[Multiple Decays Fit Parameters]]"=w214:dbl[][], "Selected ROIs Array"=w213:bool[], "IRF Array Time Axis"=w212:dbl[], "[[IRFs]]"=w211:dbl[][])
                  n60 = Unbundle By Name(w229) -> ("Parameter_Map_Plugin_Data.Parameter_Names"=w226:string[], "Parameter_Map_Plugin_Data.Parameter_Flattened_Map"=w223:dbl[][], "Parameter_Map_Plugin_Data.IRF_X"=w220:dbl[], "Parameter_Map_Plugin_Data.IRF_Y_Flattened_List"=w218:dbl[][])
                  n61 = case shown="No Error" w225 {
                    selector: w225 -> [w246 w249]
                    tunnel: [w248 w253] -> w228
                    tunnel: [w247 w254] -> w227
                    tunnel: w226 -> [w230 _]
                    tunnel: [w245 w249] -> w224
                    tunnel: w223 -> [w244 _]
                    tunnel: [w240 w252] -> w222
                    tunnel: w221 -> [w237 _]
                    tunnel: w220 -> [w236 _]
                    tunnel: [w235 w251] -> w219
                    tunnel: w218 -> [w233 _]
                    tunnel: w217 -> [w232 _]
                    tunnel: [w231 w250] -> w216
                    tunnel: w215 -> [_ w254]
                    tunnel: w214 -> [_ w253]
                    tunnel: w213 -> [_ w252]
                    tunnel: w212 -> [_ w251]
                    tunnel: w211 -> [_ w250]
                    frame No Error {
                      # "if the plugin has not provided new IRFs, use the original ones"
                      n62 = Empty Array?(array=w233) -> (empty?=w238:bool)
                      n63 = call "AlliGator Add Missing Parameter Map Parameters.vi"("Error In"=w246, "Parameter_Flattened_Map in"=w244, "Parameter Names"=w230) -> ("Error Out"=w245:errorcluster, "Parameter_Flattened_Map out"=w248:dbl[][], "[Decay Fit Parameter Name] out"=w247:T59[])  [unwired: 6 in]
                      n64 = Array Size(array=w244) -> (size(s)=w243:i32[])
                      n65 = Empty Array?(array=w236) -> (empty?=w239:bool)
                      n66 = Or(x=w239, y=w238) -> (x .or. y?=w234:bool)
                      n67 = Select(t=w237, s=w234, f=w236) -> (s? t:f=w235:dbl[])
                      n68 = Select(t=w232, s=w234, f=w233) -> (s? t:f=w231:dbl[][])
                      n69 = Index Array(array=w243) -> (element=w241:i32)  [unwired: 1 in]
                      n70 = Initialize Array(TRUE ("Selected"), w241) -> (w240:bool[])
                    }
                    frame Error {
                    }
                  }
                  n71 = in-place-cluster #8("[Decay Fit Parameter Names]"=w227, "[[Multiple Decays Fit Parameters]]"=w228, "Selected ROIs Array"=w222, "IRF Array Time Axis"=w219, "[[IRFs]]"=w216) -> (w208:T23)
                }
                n72 = in-place-dvr #7(w208) -> (w202:refnum<data-value>)  [unwired: 1 out]
              }
            }
            frame "", Default {
              n73 = in-place {
                in-place-border: w262 -> [w273]
                in-place-border: w261 -> [w271]
                in-place-border: [w270] -> w260
                in-place-border: w259 -> [w269]
                in-place-border: [w268] -> w258
                in-place-border: w257 -> [w267]
                in-place-border: w256 -> [w266]
                in-place-border: [w265] -> w255
                n74 = in-place-dvr #9(w264) -> (w274:T23)  [unwired: 1 out]
                n75 = in-place {
                  in-place-border: w273 -> [w285]
                  in-place-border: w271 -> [w291]
                  in-place-border: [w290] -> w270
                  in-place-border: w269 -> [w287]
                  in-place-border: [w278] -> w268
                  in-place-border: w267 -> [w281]
                  in-place-border: w266 -> [w280]
                  in-place-border: [w275] -> w265
                  n76 = in-place-cluster #10(w274) -> ("[Map Set Names]"=w279:string[], "[Parameter Maps]"=w289:T61[])
                  n77 = Unbundle By Name(w285) -> ("Parameter_Map_Plugin_Data"=w284:T18, "Parameter_Map_Plugin_Data.IRF_X"=w283:dbl[], "Parameter_Map_Plugin_Data.IRF_Y_Flattened_List"=w282:dbl[][])
                  n78 = call "AlliGator Build Python Plugin Parameter Map.vi"("error in (no error)"=w291, "Parameter_Map_Data"=w284, "Function Display Name"=w287, "[Map Set Names] in"=w279) -> ("error out"=w290:errorcluster, "New Parameter Names"=w277:string[], "Parameter Map out"=w286:T61, "[Map Set Names] out"=w276:string[], "Message"=w278:string)  [unwired: 3 in]
                  n79 = case shown="No Error" w290 {
                    tunnel: w289 -> [w309 w310]
                    tunnel: [w308 w310] -> w288
                    tunnel: w286 -> [w307 _]
                    tunnel: w283 -> [w303 _]
                    tunnel: w282 -> [w302 _]
                    tunnel: w281 -> [w301 _]
                    tunnel: w280 -> [w300 _]
                    tunnel: w277 -> [w295 _]
                    tunnel: w276 -> [w293 _]
                    tunnel: [w294 _] -> w275
                    frame No Error {
                      # "if the plugin has not provided new IRFs, use the original ones"
                      n80 = Empty Array?(array=w302) -> (empty?=w305:bool)
                      n81 = Empty Array?(array=w303) -> (empty?=w306:bool)
                      n82 = Or(x=w306, y=w305) -> (x .or. y?=w304:bool)
                      n83 = Delete From Array(array=w293) -> (deleted portion=w292:string)  [unwired: 2 in, 1 out]
                      n84 = Select(t=w301, s=w304, f=w303) -> (s? t:f=w298:dbl[])
                      n85 = Select(t=w300, s=w304, f=w302) -> (s? t:f=w297:dbl[][])
                      n86 = Bundle By Name(cluster=T22 {"New Parameter Set Name"="", "Parameter Map Names"=[]} ("New Parameter Map Set"), "New Parameter Set Name"=w292, "Parameter Map Names"=w295) -> (w294:T22)
                      n87 = Bundle By Name(cluster=w307, "IRF Array Time Axis"=w298, "[[IRFs]]"=w297) -> (w299:T61)
                      n88 = Build Array (concatenate)(w309, w299) -> (w308:T61[])
                    }
                    frame Error {
                    }
                  }
                  n89 = in-place-cluster #10("[Map Set Names]"=w276, "[Parameter Maps]"=w288) -> (w272:T23)
                }
                n90 = in-place-dvr #9(w272) -> (w263:refnum<data-value>)  [unwired: 1 out]
              }
            }
          }
        }
        frame 2 {
          # "Plots output"
          n91 = call "AlliGator Python Plugin Data to Graph v1.1.vi"("AlliGator Ctrl Refnums"=w311, "error in (no error)"=w315, "Output Destination"=w313, "Plugin_Data"=w314) -> ("Message"=w312:string)  [unwired: 6 in, 1 out]
        }
      }
    }
    frame Error {
    }
  }
  "Data Value Reference out" <- w39
  "Variant data out" <- w13
  n92 = call "High Resolution Timing.vi"("relative seconds (NaN)"=w15, "Error In"=w69) -> ("elapsed (relative) seconds"=w14:dbl, "Error Out"=w16:errorcluster)  [unwired: 15 in, 1 out]
  n93 = Format Into String(format string="\\n%s\\n%s", initial string=w48, error in=w16, w21, w20) -> (resulting string=w56:string, error out=w55:errorcluster)
  n94 = Format Into String(format string=" used as %s\nCPU: %#g s", initial string=w56, error in=w55, w6, w14) -> (resulting string=→"Message":string, error out=w54:errorcluster)
  n95 = call "Alligator Variables Storage.vi"("Get(F)/Set"=w51, "AlliGator Variable"=w52, "Error In"=w54, "Data in"=w51) -> ("Error Out"=→"error out":errorcluster)  [unwired: 5 in, 2 out]
